vi "Watchdog Globals.vi"() -> ()   [LabVIEW 2014]
panel:
  in  "Control Inputs Valid":bool
  in  "Emergency Safe":bool
  in  "Watchdog Safe":bool
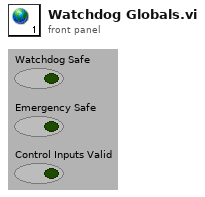
[diagram p1: front panel]
diagram:
